vi "Buzzer Pressed.vi"(8 "error in (no error)":errorcluster, 11 "Sounds in":refnum<class "Sounds.lvclass">) -> (0 "error out":errorcluster, 3 "Sounds out":refnum<class "Sounds.lvclass">)   [LabVIEW 2024]
uses:
  Sounds.lvclass
panel:
  out "error out 2":errorcluster
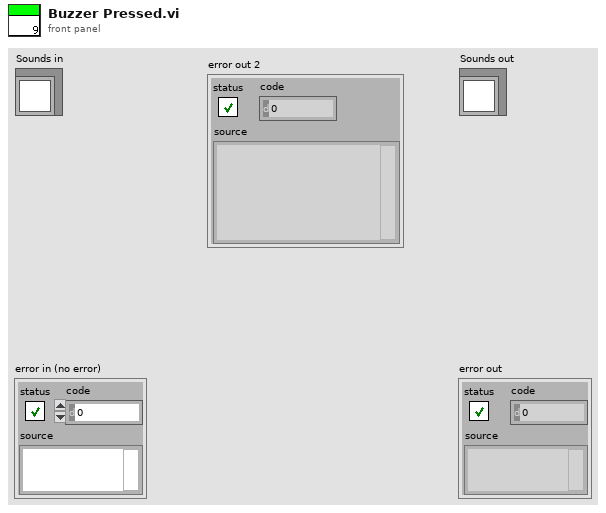
[diagram p1: front panel]
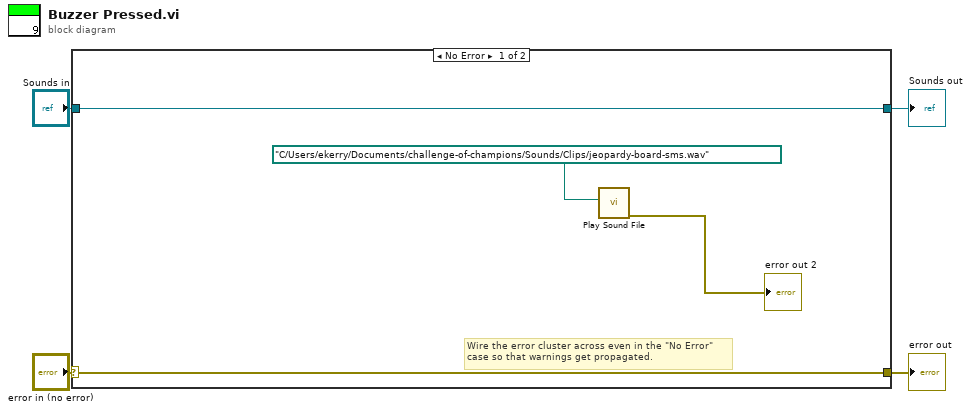
[diagram p0: block diagram]
diagram:
  n1 = case shown="No Error" "error in (no error)" {
    selector: "error in (no error)" -> [w7 w10]
    tunnel: [w7 w10] -> w3
    tunnel: [w8 w9] -> w1
    tunnel: "Sounds in" -> [w8 w9]
    frame No Error {
      # "Wire the error cluster across even in the \"No Error\"\ncase so that warnings get propagated."
      n2 = call <vilib>:"Play Sound File.vi"("path"=path "C:/Users/ekerry/Documents/challenge-of-champions/Sounds/Clips/jeopardy-board-sms.wav") -> ("error out"=→"error out 2":errorcluster)  [unwired: 9 in, 1 out]
    }
    frame Error {
    }
  }
  "error out" <- w3
  "Sounds out" <- w1
